vi "SimpleHEAT3.vi"() -> ()   [LabVIEW 2020]
uses:
  Control 2.ctl
  rga_lv_85/SRSRGA85.llb/SRSRGAo RefNum.ctl
  <vilib>/Utility/miscctls.llb/LVRowAndColumnTypeDef.ctl
  <vilib>/Modbus/master/Create Master Instance (TCP).vi
  <vilib>/Utility/config.llb/Read Key (String).vi
  <vilib>/Utility/config.llb/Write Key (String).vi
  <vilib>/Modbus/master/Modbus Master.lvclass
  <vilib>/Utility/config.llb/NI_LVConfig.lvlib
panel:
  in  "stop":bool
  out "Remote:":bool
  out "heat_LastData":dbl[](array[numeric])
  out "HEAT start time":timestamp=timestamp(3621395400.2120705 s since 1904-01-01)
  out "Boolean":T1=TRUE
  out "stopped_loops":bool=TRUE
  in  "Tab Control":T2(tab)
  out "Uc Act.: 2":dbl caption="Uc Act.:" format="%#_g V"
  out "Ic Act.: 2":dbl caption="Ic Act.:" format="%#_g A"
  out "Ue Act.: 2":dbl caption="Ue Act.:" format="%#_g V"
  out "Ie Act.: 2":dbl caption="Ie Act.:" format="%#_g mA"
  out "Text Ring 6":u16(ring) items=["K"=1, "C"=0]
  out "Text Ring 5":u16(ring) items=["C/s", "C/m", "C/h"]
  out "Act. Ramp:":dbl=1.0
  in  "Regulation TYpe":bool caption="Regulation Type:"
  in  "Target Ue [V]:":dbl=500.0
  in  "Target Ic [A]:":dbl=2.0
  in  "PID Output:":bool caption="PID Output Signal:"
  in  "Heating Mode:":bool
  out "Text Ring 3":u16(ring) items=["C/s", "C/m", "C/h"]
  out "Interlock:":bool
  out "Operate:":bool
  out "Text Ring":u16(ring) items=["K"=1, "C"=0]
  in  "OperateButton":bool caption="Operate:"
  out "Act. Temp:":dbl=24.100000000000023
  out "Act. P":dbl=100.0
  out "Act. I":dbl=50.0
  out "Act. D":dbl=1.0
  in  "Target Temp:":dbl=10.0
  in  "Target Ramp:":dbl=1.0
  out "Act. Setpoint:":dbl=21.55000000000001
  out "Text Ring 2":u16(ring) items=["K"=1, "C"=0]
  out "RES active:":bool
  out "EB active:":bool
  in  "Ramp unit:":u16(ring)=1 items=["/s", "/m", "/h"]
  in  "Temp. unit:":u16(ring) items=["K"=1, "C"=0]
  in  "Channel:":u16(ring)=7 items=["D1"=9, "D2"=11, "RTD"=13, "TC1"=5, "TC2"=7]
  in  "clean":bool
  out "Operate status::":bool[](array[boolean])=[FALSE, FALSE, FALSE, FALSE, FALSE, TRUE, TRUE, TRUE, FALSE, FALSE, FALSE, TRUE, FALSE, FALSE, FALSE, FALSE]
  out "Uc Act.:":dbl
  out "Ic Act.:":dbl
  out "Uc Act.:":dbl
  out "Ic Act.:":dbl
  out "Ue Act.:":dbl
  out "Ie Act.:":dbl
  in  "Ie limit [mA]:":dbl
  in  "Ue limit [V]:":dbl
  in  "Ic limit [A]:":dbl
  in  "Uc limit [V]:":dbl
  in  "Ic limit:1":dbl caption="Ic limit [A]:"
  in  "Uc limit:1":dbl caption="Uc limit [V]:"
  out "New D:":dbl=1.0
  out "New I:":dbl=50.0
  out "New P:":dbl=100.0
  in  "PID auto tab":string[][](table)
  in  "PID manual setting":string[][](table)=[["100", "50", "1"]]
  in  "Auto PID control:":bool=TRUE
  out "New PID request":bool
  out "Connected:":bool=TRUE
  in  "Reconect":bool
  out "Comunication error:":bool
  out "Loop time:":u32=499
  in  "Lock Button":bool
  in  "Address:":string="192.168.201.50"
  out "error out":T3
  # "RES:"
  # "EB:"
  # "EB:"
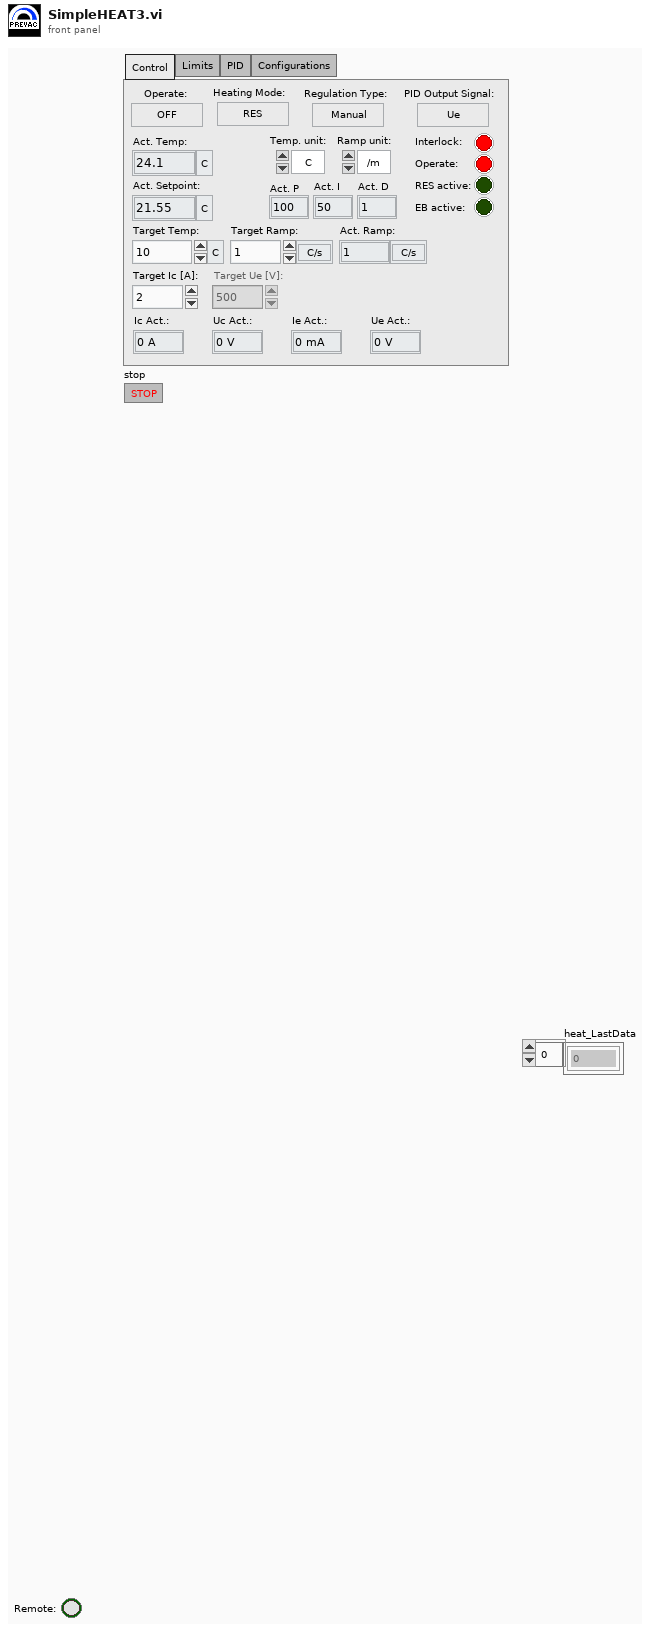
[diagram p1: front panel]
types:
  T1 = typedef "Control 2.ctl" = bool
  T2 = enum32{"Control", "Limits", "PID", "Configurations"}
  T3 = cluster{"Status:":bool, "Code:":i32, "source":string}
  T4 = typedef "SRSRGAo RefNum.ctl" = u16
  T5 = typedef "LVRowAndColumnTypeDef.ctl" = cluster{"Row":i32, "Column":i32}
  T6 = enum8{"Enabled", "Disabled", "Disabled and Grayed Out"}
  T7 = typedef "NI_LVConfig.lvlib/Config Data RefNum.ctl" = refnum<k1>
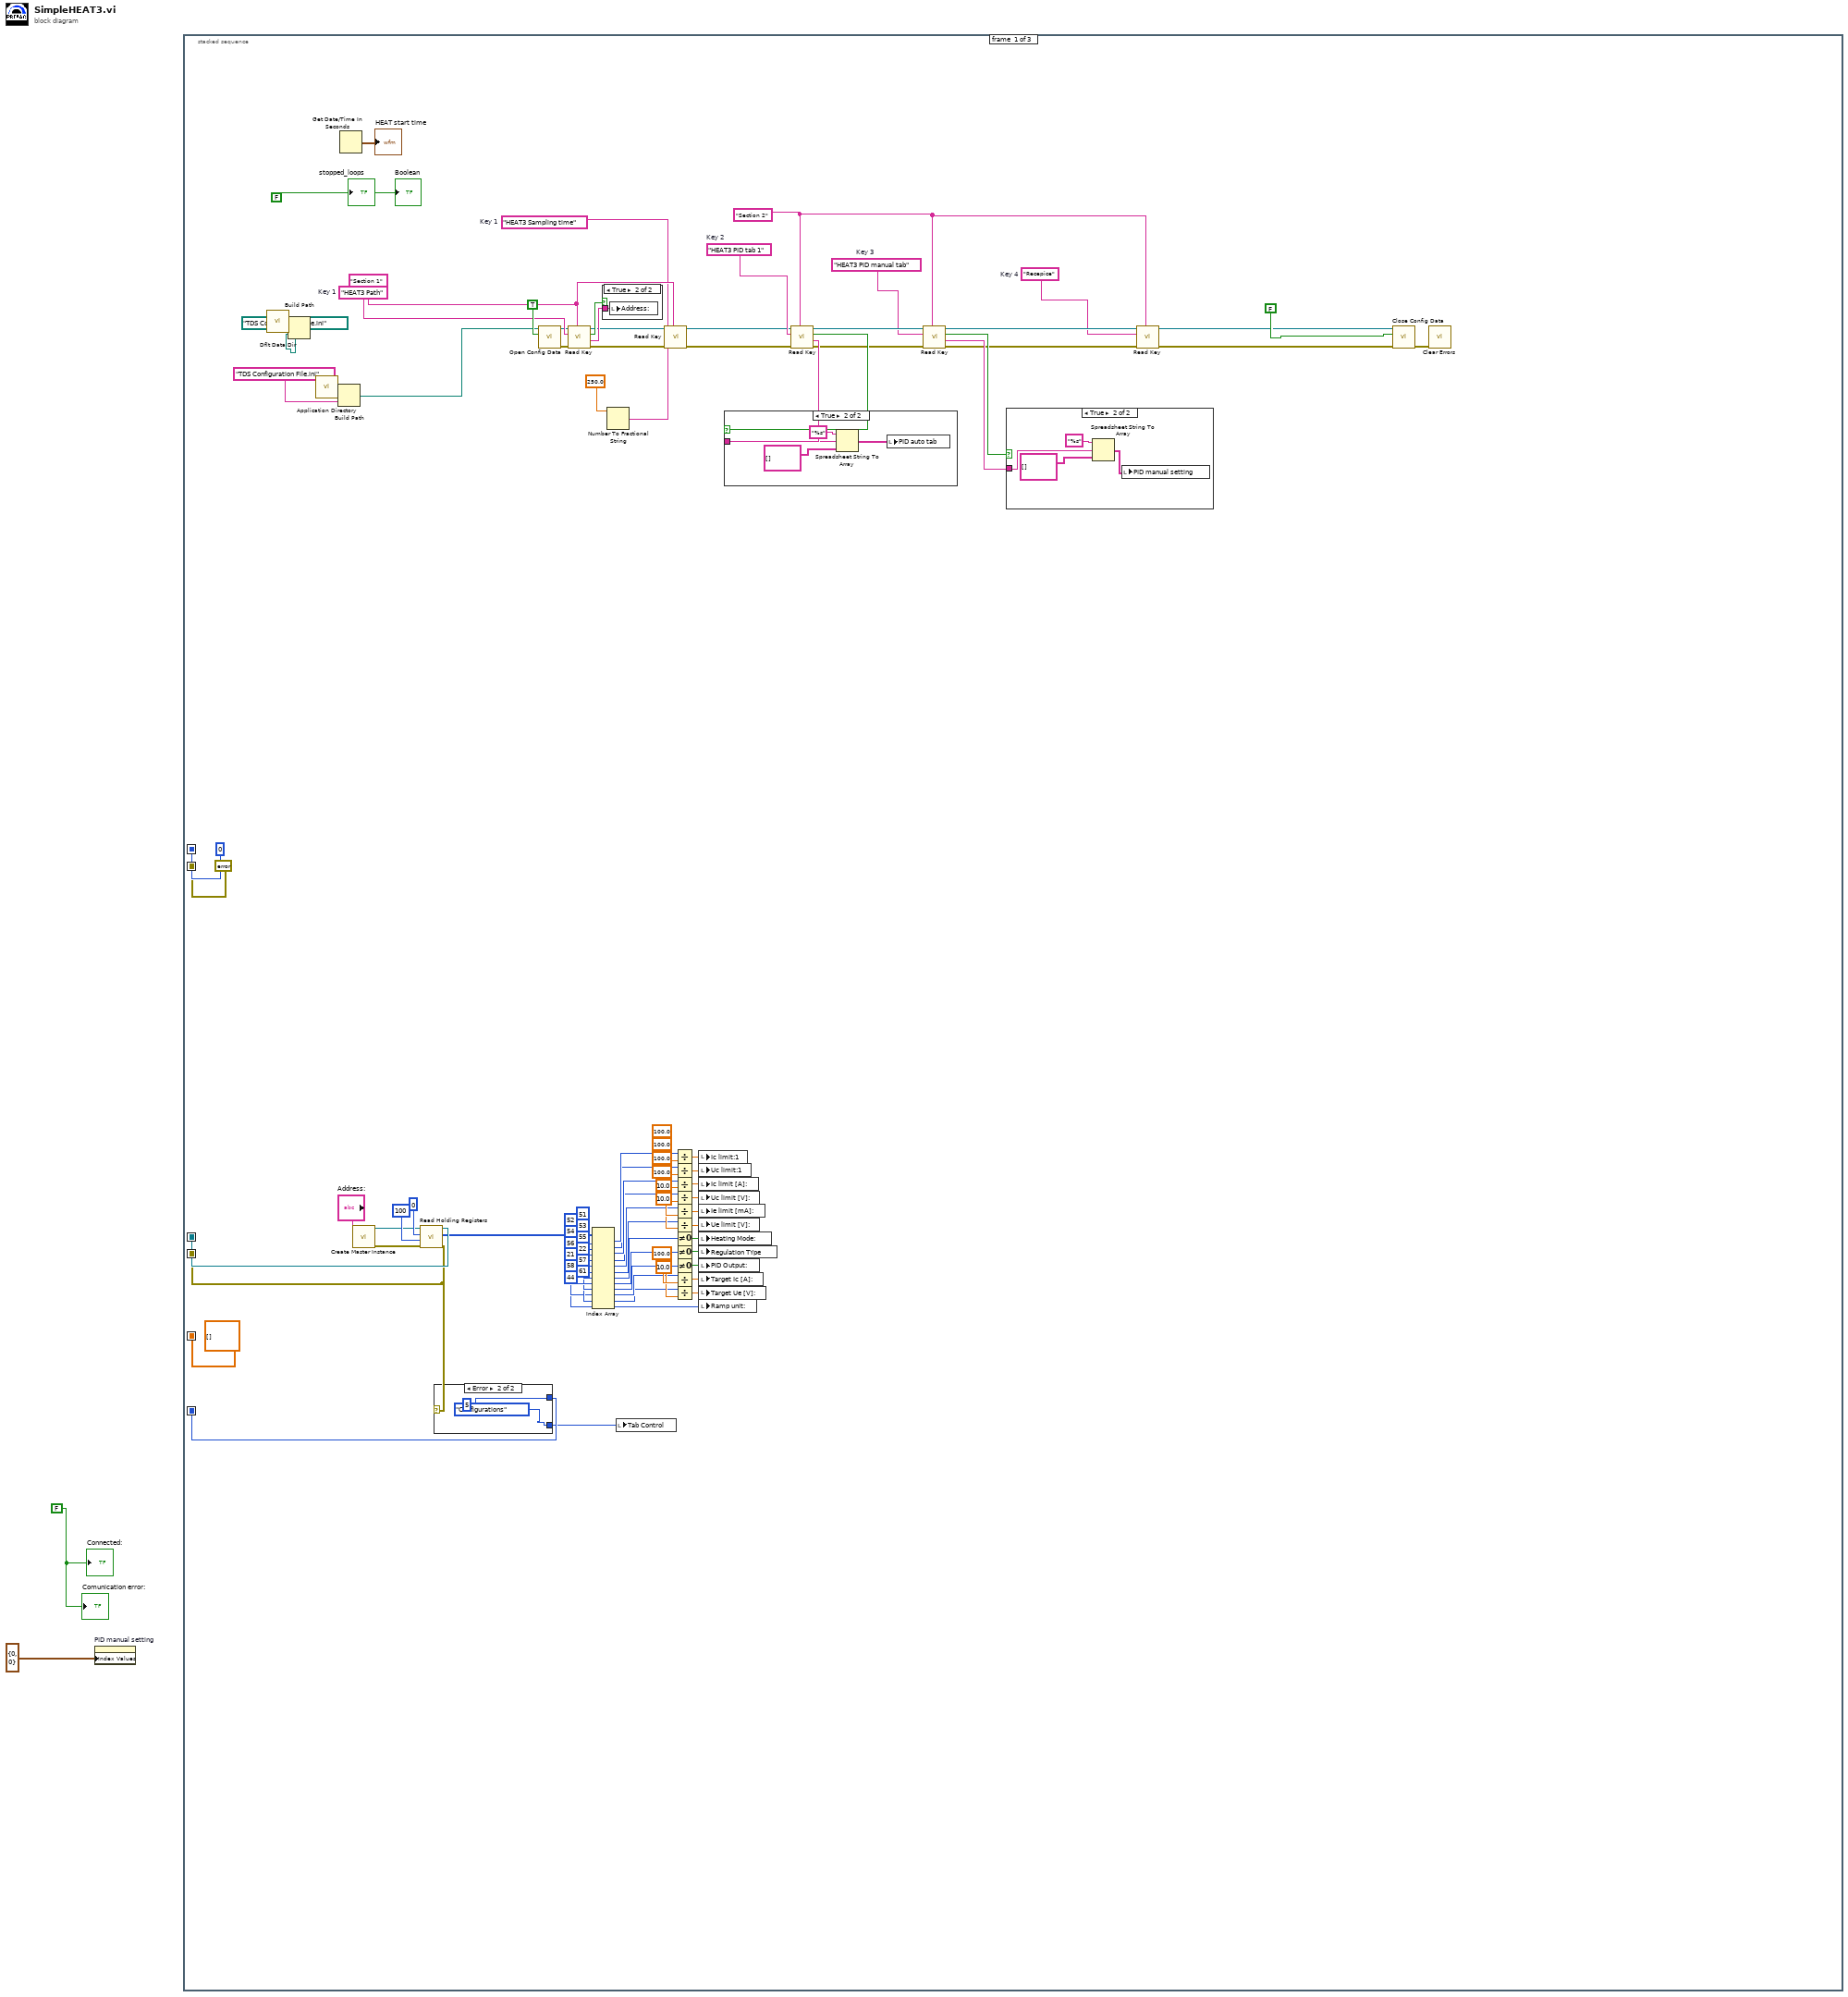
[diagram p0: block diagram]
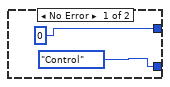
[diagram p4: hidden frame]
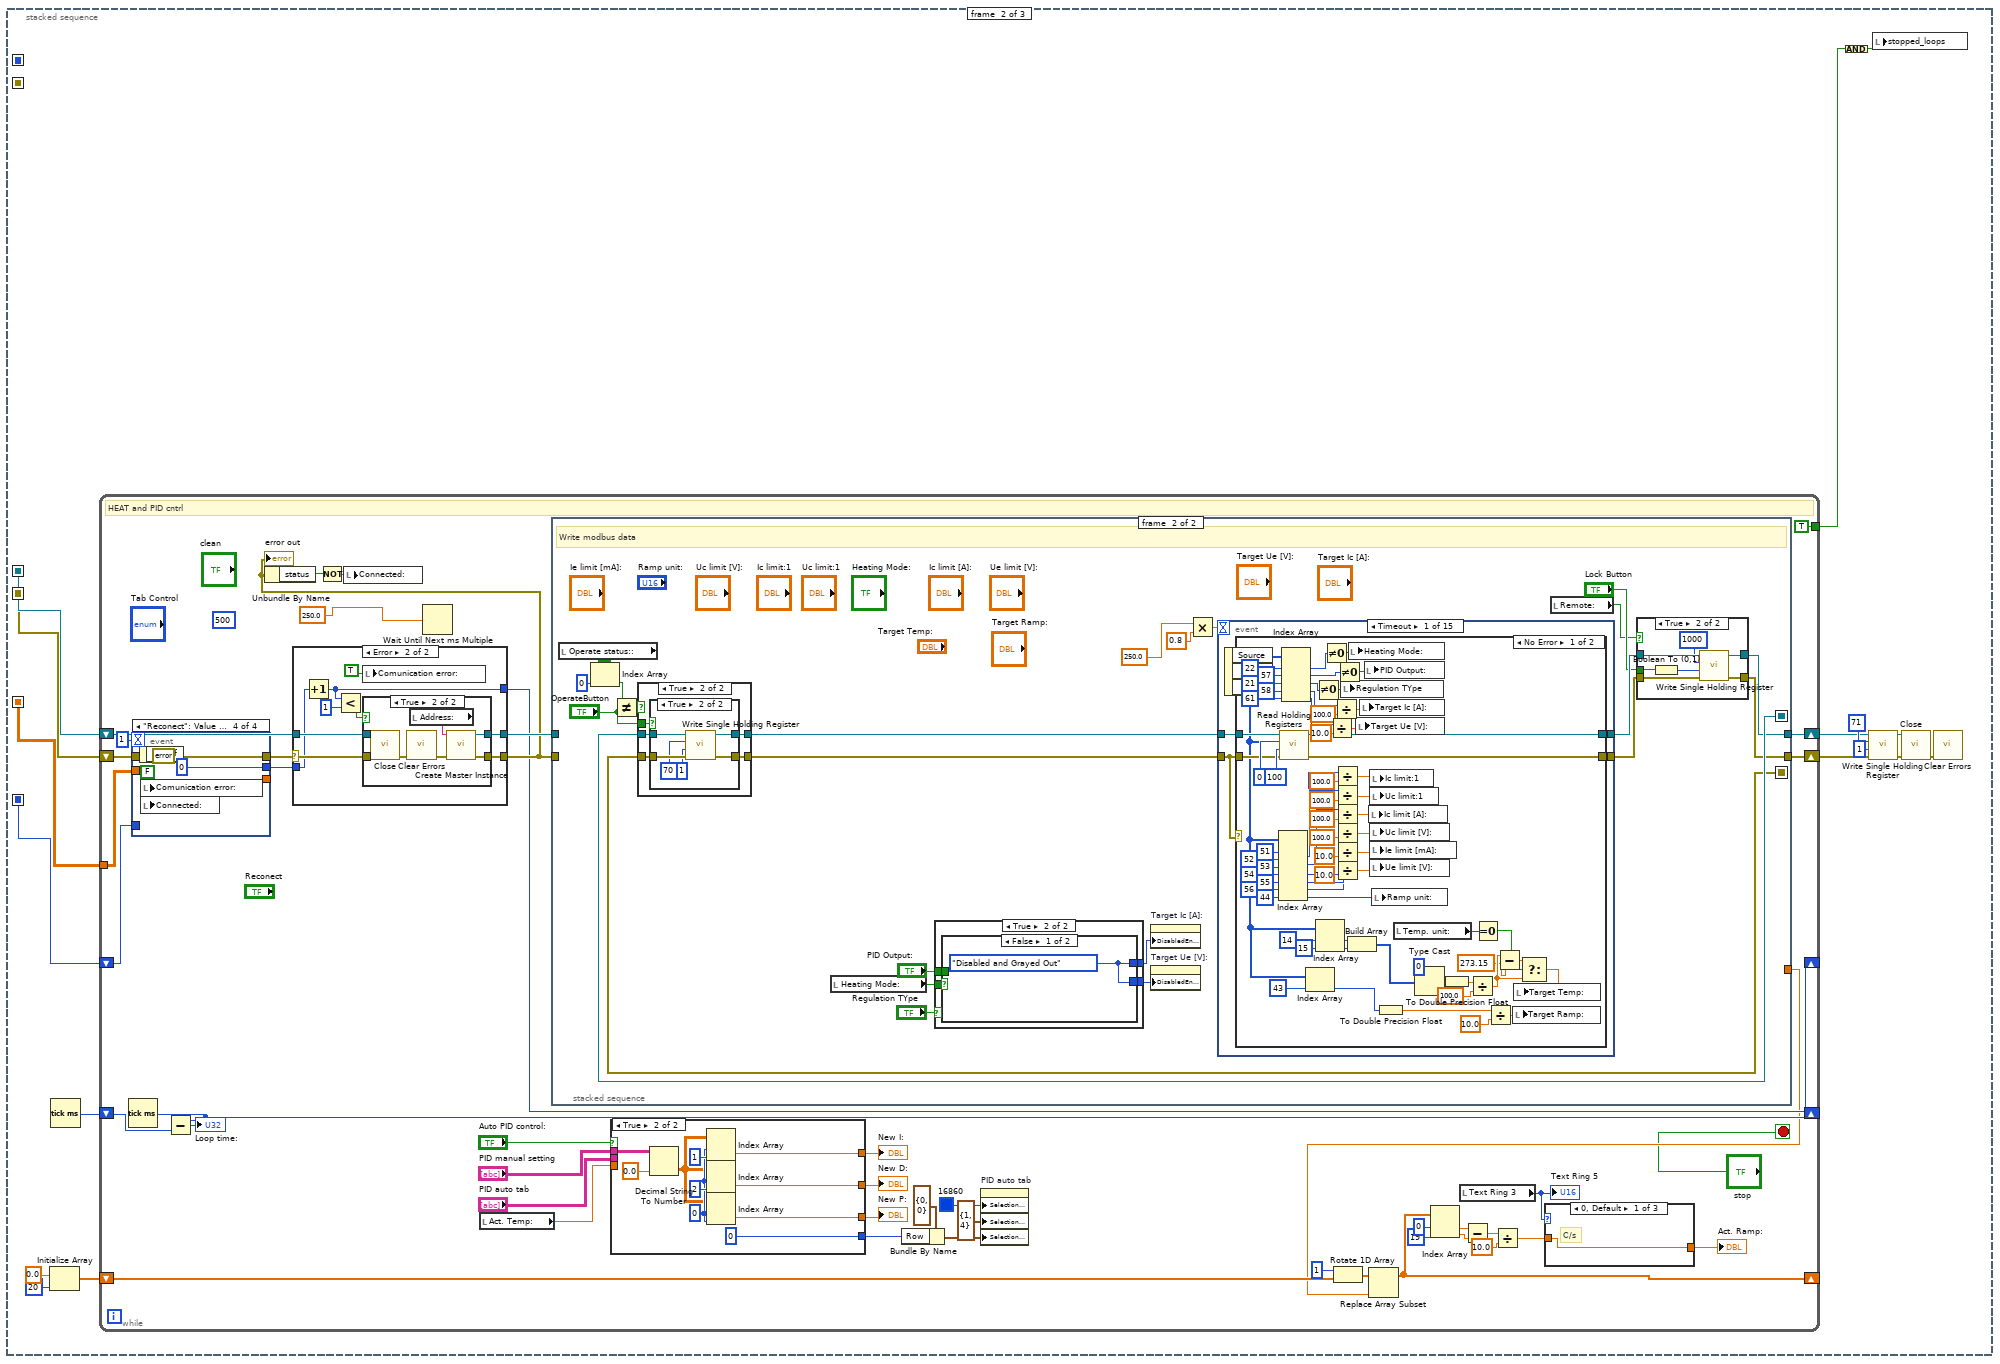
[diagram p6: hidden frame]
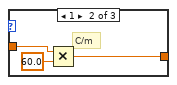
[diagram p7: hidden frame]
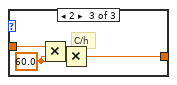
[diagram p8: hidden frame]
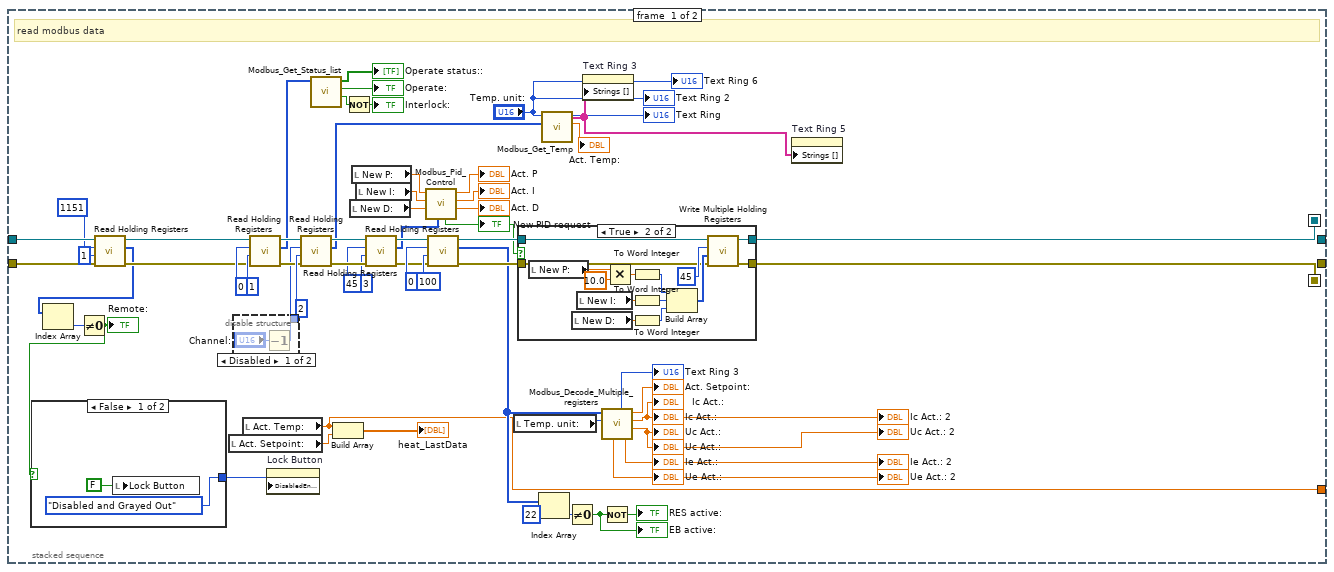
[diagram p9: hidden frame]
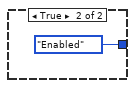
[diagram p10: hidden frame]
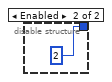
[diagram p11: hidden frame]
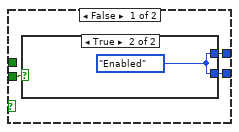
[diagram p14: hidden frame]
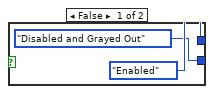
[diagram p15: hidden frame]
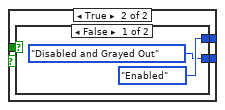
[diagram p16: hidden frame]
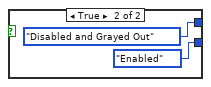
[diagram p17: hidden frame]
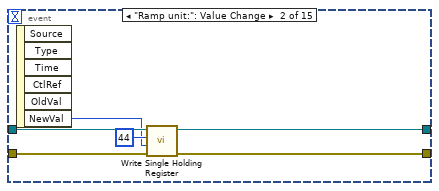
[diagram p19: hidden frame]
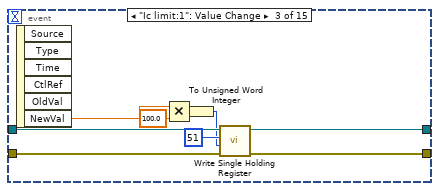
[diagram p20: hidden frame]
diagram:
  w2 = FALSE ("Connected:")
  n1 = property on="PID manual setting" class="Tbl (strict)"("Index Values"=cluster{"Row":u32, "Column":u32} {"Row"=0, "Column"=0}) -> ()  [unwired: 2 in, 2 out]
  n2 = stacked-sequence {
    seq-local: [w80 _ _] -> [_ w124 _]
    seq-local: [w33 _ _] -> [_ w123 _]
    seq-local: [dbl[][] [] _ _] -> [_ w110 _]
    seq-local: [T4 0 ("SRSRGA Refnum") _ _] -> [_ _ _]
    seq-local: [errorcluster {"status"=FALSE, "code"=0, "source"=""} ("error out") _ _] -> [_ _ _]
    seq-local: [w32 _ _] -> [_ w115 _]
    frame #0 {
      w9 = "HEAT3 Sampling time"  # Key 1
      w19 = "Recepice"  # Key 4
      w26 = "HEAT3 PID manual tab"  # Key 3
      w31 = "HEAT3 PID tab 1"  # Key 2
      w18 = "Section 2" ("section")
      w87 = "HEAT3 Path"  # Key 1
      w10 = "Section 1" ("section")
      w17 = FALSE ("Boolean")
      n3 = call <vilib>:"Dflt Data Dir.vi"() -> ("App:Default Data Directory"=w92:path)
      n4 = Build Path(base path=w92, name or relative path=path "TDS Configuration File.ini" ("default name")) -> ()  [unwired: 1 out]
      n5 = call <vilib>:"Application Directory.vi"() -> ("Application Directory"=w14:path)
      n6 = Build Path(base path=w14, name or relative path="TDS Configuration File.ini") -> (appended path=w13:path)
      n7 = Get Date/Time In Seconds() -> (seconds since 1Jan1904=→"HEAT start time":timestamp)
      n8 = call-poly <vilib>:"Create Master Instance.vi"("address"="Address:") -> ("error out"=w81:errorcluster, "TCP master instance"=w82:refnum<class "Modbus Master.lvclass">)  [unwired: 9 in]
      n9 = call-dynamic "Read Holding Registers.vi"("error in (no error)"=w81, "number of holding registers"=u16 100, "starting address"=u16 0, "Modbus master in"=w82) -> ("error out"=w33:errorcluster, "register values"=w75:u16[], "Modbus master out"=w80:refnum<class "Modbus Master.lvclass">)  [unwired: 5 in]
      n10 = case shown="Error" w33 {
        tunnel: [0 5] -> w32
        tunnel: [T2."Control" ("Tab Control") T2."Configurations" ("Tab Control")] -> w3
        frame No Error {
        }
        frame Error {
        }
      }
      n11 = call <vilib>:"Open Config Data.vi"("create file if necessary (T)"=TRUE ("create file if necessary? (T)"), "configuration file path"=w13) -> ("error out"=w85:errorcluster, "refnum"=w86:T7)  [unwired: 7 in, 1 out]
      n12 = call-poly <vilib>:"Read Key.vi"("section"=w10, "error in (no error)"=w85, "key"=w87, "refnum"=w86) -> ("error out"=w6:errorcluster, "value"=w89:string, "found?"=w88:bool, "refnum out"=w8:T7)  [unwired: 2 in, 2 out]
      n13 = Index Array(array=w75, index #1=51 ("index"), index #2=52 ("index"), index #3=53 ("index"), index #4=54 ("index"), index #5=55 ("index"), index #6=56 ("index"), index #7=22 ("index"), index #8=21 ("index"), index #9=57 ("index"), index #10=58 ("index"), index #11=61 ("index"), index #12=44 ("index")) -> (element #1=w66:u16, element #2=w65:u16, element #3=w64:u16, element #4=w52:u16, element #5=w63:u16, element #6=w51:u16, element #7=w55:u16, element #8=w4:u16, element #9=w44:u16, element #10=w37:u16, element #11=w36:u16, element #12=w34:u16)
      n14 = case shown="True" w88 {
        tunnel: w89 -> [_ w108]
        frame False {
        }
        frame True {
          n15 = local write "Address:"(w108) -> ()
        }
      }
      n16 = Number To Fractional String(number=250.0) -> (F-format string=w11:string)  [unwired: 3 in]
      n17 = local write "Tab Control"(w3) -> ()
      n18 = call-poly <vilib>:"Read Key.vi"("section"=w10, "error in (no error)"=w6, "default value"=w11, "key"=w9, "refnum"=w8) -> ("error out"=w5:errorcluster, "refnum out"=w7:T7)  [unwired: 1 in, 4 out]
      n19 = Divide(x=w66, y=100.0) -> (x/y=w62:dbl)
      n20 = Divide(x=w65, y=100.0) -> (x/y=w61:dbl)
      n21 = Divide(x=w64, y=100.0) -> (x/y=w60:dbl)
      n22 = Divide(x=w52, y=100.0) -> (x/y=w59:dbl)
      n23 = Divide(x=w63, y=10.0) -> (x/y=w58:dbl)
      n24 = Divide(x=w51, y=10.0) -> (x/y=w57:dbl)
      n25 = Not Equal To 0?(x=w55) -> (x != 0?=w54:bool)
      n26 = Not Equal To 0?(x=w4) -> (x != 0?=w48:bool)
      n27 = Not Equal To 0?(x=w44) -> (x != 0?=w47:bool)
      n28 = Divide(x=w37, y=100.0) -> (x/y=w41:dbl)
      n29 = Divide(x=w36, y=10.0) -> (x/y=w40:dbl)
      n30 = local write "Ic limit:1"(w62) -> ()
      n31 = local write "Uc limit:1"(w61) -> ()
      n32 = local write "Ic limit [A]:"(w60) -> ()
      n33 = local write "Uc limit [V]:"(w59) -> ()
      n34 = local write "Ie limit [mA]:"(w58) -> ()
      n35 = local write "Ue limit [V]:"(w57) -> ()
      n36 = local write "Heating Mode:"(w54) -> ()
      n37 = local write "Regulation TYpe"(w48) -> ()
      n38 = local write "PID Output:"(w47) -> ()
      n39 = local write "Target Ic [A]:"(w41) -> ()
      n40 = local write "Target Ue [V]:"(w40) -> ()
      n41 = local write "Ramp unit:"(w34) -> ()
      n42 = call-poly <vilib>:"Read Key.vi"("section"=w18, "error in (no error)"=w5, "key"=w31, "refnum"=w7) -> ("error out"=w27:errorcluster, "value"=w29:string, "found?"=w30:bool, "refnum out"=w28:T7)  [unwired: 2 in, 2 out]
      n43 = case shown="True" w30 {
        tunnel: w29 -> [_ w103]
        frame False {
        }
        frame True {
          n44 = Spreadsheet String To Array(format string="%s", spreadsheet string=w103, array type (2D Dbl)=string[][] [] ("PID auto tab")) -> (array=w100:string[][])  [unwired: 1 in]
          n45 = local write "PID auto tab"(w100) -> ()
        }
      }
      n46 = call-poly <vilib>:"Read Key.vi"("section"=w18, "error in (no error)"=w27, "key"=w26, "refnum"=w28) -> ("error out"=w23:errorcluster, "value"=w24:string, "found?"=w25:bool, "refnum out"=w21:T7)  [unwired: 2 in, 2 out]
      n47 = case shown="True" w25 {
        tunnel: w24 -> [_ w97]
        frame False {
        }
        frame True {
          n48 = Spreadsheet String To Array(format string="%s", spreadsheet string=w97, array type (2D Dbl)=string[][] [] ("PID auto tab")) -> (array=w96:string[][])  [unwired: 1 in]
          n49 = local write "PID manual setting"(w96) -> ()
        }
      }
      n50 = call-poly <vilib>:"Read Key.vi"("section"=w18, "error in (no error)"=w23, "key"=w19, "refnum"=w21) -> ("error out"=w22:errorcluster, "refnum out"=w20:T7)  [unwired: 2 in, 4 out]
      n51 = call <vilib>:"Close Config Data.vi"("error in (no error)"=w22, "write file if changed (T)"=FALSE ("write configuration file? (T)"), "refnum"=w20) -> ("error out"=w16:errorcluster)  [unwired: 8 out]
      n52 = call <vilib>:"Clear Errors.vi"("error in (no error)"=w16) -> ()  [unwired: 5 in, 2 out]
      "stopped_loops" <- w17
      "Boolean" <- w17
    }
    frame #1 {
      n53 = Initialize Array(0.0 ("element"), 20 ("dimension size")) -> (w112:dbl[])
      n54 = Tick Count (ms)() -> (millisecond timer value=w111:u32)
      n55 = while {
        tunnel: [TRUE] -> w116
        shift-right: [w156] -> w119
        shift-left: w123 -> [w149]
        shift-right: [w159] -> w120
        shift-left: w124 -> [w158]
        shift-right: [w153] -> _
        shift-left: w111 -> [w152]
        shift-right: [w142] -> _
        shift-left: w115 -> [w147]
        tunnel: w110 -> [w154]
        shift-right: [w138] -> _
        shift-left: w112 -> [w141]
        stop <- "stop" stop-if-true
        (unwired) u32 500 ("millisecond multiple")
        # "HEAT and PID cntrl"
        n56 = Tick Count (ms)() -> (millisecond timer value=w153:u32)
        n57 = event shown="[3] \"Reconect\": Value Change" {
          selector: _ -> [_ _ _ _]
          dyn-events: _ -> [_ _ _ _]
          timeout: 1 -> [_ _ _ _]
          tunnel: w154 -> [w540 _ _ _]
          tunnel: [w538 dbl[][] [] _ _] -> _
          tunnel: [w537 w543 errorcluster {"status"=TRUE, "code"=0, "source"="Connect to\nnew IP addres"} ("error constant") errorcluster {"status"=TRUE, "code"=0, "source"="Rconnecting"} ("error constant")] -> w148
          tunnel: w149 -> [w537 w543 _ _]
          tunnel: [w536 w542 0 0] -> w146
          tunnel: w147 -> [w536 w542 _ _]
          event Timeout {
            n58 = event-data() -> ()  [unwired: 1 in, 1 out]
            n59 = Select(t=w540, s=FALSE ("build array of data?"), f=dbl[][] []) -> (s? t:f=w538:dbl[][])
          }
          event "clean": Value Change {
            n60 = event-data() -> ()  [unwired: 1 in, 1 out]
            n61 = Get Date/Time In Seconds() -> (seconds since 1Jan1904=w544:timestamp)
            n62 = local write "HEAT start time"(w544) -> ()
            n63 = local write "clean"(FALSE ("clc graph")) -> ()
          }
          event "Address:": Value Change {
            n64 = event-data() -> ()  [unwired: 1 in, 1 out]
          }
          event "Reconect": Value Change {
            w549 = FALSE ("Connected:")
            n65 = event-data() -> ()  [unwired: 1 in, 1 out]
            n66 = local write "Comunication error:"(w549) -> ()
            n67 = local write "Connected:"(w549) -> ()
          }
        }
        n68 = Subtract(x=w153, y=w152) -> (x-y=→"Loop time:":u32)
        n69 = case shown="Error" w148 {
          selector: w148 -> [w556 w565]
          tunnel: [w556 w562] -> w144
          tunnel: w158 -> [w555 w564]
          tunnel: [w555 w563] -> w157
          tunnel: w146 -> [_ w560]
          tunnel: [0 w559] -> w142
          frame No Error {
            w552 = FALSE
            n70 = Not(x=w552) -> (.not. x?=w553:bool)
            n71 = local write "Comunication error:"(w552) -> ()
            n72 = local write "Connected:"(w553) -> ()
          }
          frame Error {
            n73 = Increment(x=w560) -> (x+1=w559:i32)
            n74 = Less?(x=w559, y=1) -> (x < y?=w558:bool)
            n75 = local write "Comunication error:"(TRUE) -> ()
            n76 = case shown="True" w558 {
              tunnel: w565 -> [w566 w574]
              tunnel: w564 -> [w567 w573]
              tunnel: [w567 w571] -> w563
              tunnel: [w566 w570] -> w562
              frame False {
              }
              frame True {
                n77 = call-dynamic "Close.vi"("error in (no error)"=w574, "Modbus master in"=w573) -> ("error out"=w569:errorcluster)  [unwired: 9 in]
                n78 = call <vilib>:"Clear Errors.vi"("error in (no error)"=w569) -> ("error out"=w568:errorcluster)  [unwired: 5 in, 1 out]
                n79 = local read "Address:"() -> (w572:string)
                n80 = call-poly <vilib>:"Create Master Instance.vi"("error in (no error)"=w568, "address"=w572) -> ("error out"=w570:errorcluster, "TCP master instance"=w571:refnum<class "Modbus Master.lvclass">)  [unwired: 8 in]
              }
            }
          }
        }
        "error out" <- w144
        n81 = Unbundle By Name(w144) -> ("status"=w145:bool)
        n82 = Not(x=w145) -> (.not. x?=w143:bool)
        n83 = local write "Connected:"(w143) -> ()
        n84 = Wait Until Next ms Multiple(millisecond multiple=250.0 ("y")) -> ()  [unwired: 1 out]
        n85 = local read "Act. Temp:"() -> (w160:dbl)
        n86 = stacked-sequence {
          seq-local: [w200 _] -> [_ w279]
          seq-local: [w199 _] -> [_ w278]
          tunnel: w157 -> [w198 _]
          tunnel: w144 -> [w197 _]
          tunnel: [_ w271] -> w159
          tunnel: [_ w269] -> w156
          tunnel: [w188 _] -> w128
          frame #0 {
            # "read modbus data"
            n87 = call-dynamic "Read Holding Registers.vi"("error in (no error)"=w197, "number of holding registers"=u16 1, "starting address"=u16 1151, "Modbus master in"=w198) -> ("error out"=w195:errorcluster, "register values"=w189:u16[], "Modbus master out"=w196:refnum<class "Modbus Master.lvclass">)  [unwired: 5 in]
            n88 = Index Array(array=w189) -> (element=w190:u16)  [unwired: 1 in]
            n89 = Not Equal To 0?(x=w190) -> (x != 0?=w191:bool)
            "Remote:" <- w191
            n90 = case shown="False" w191 {
              tunnel: [T6."Disabled and Grayed Out" ("Disabled") T6."Enabled" ("Disabled")] -> w192
              frame False {
                n91 = local write "Lock Button"(FALSE ("Lock Button")) -> ()
              }
              frame True {
              }
            }
            n92 = local read "Act. Setpoint:"() -> (w213:dbl)
            n93 = disable-structure shown="Disabled" {
              disable-tunnel: [w243 u16 2] -> w218
              frame Disabled {
                n94 = Decrement(x="Channel:") -> (x-1=w243:u16)
              }
              frame Enabled {
              }
            }
            n95 = local read "Act. Temp:"() -> (w188:dbl)
            n96 = call-dynamic "Read Holding Registers.vi"("error in (no error)"=w195, "number of holding registers"=u16 1, "starting address"=u16 0, "Modbus master in"=w196) -> ("error out"=w231:errorcluster, "register values"=w206:u16[], "Modbus master out"=w232:refnum<class "Modbus Master.lvclass">)  [unwired: 5 in]
            n97 = property on="Lock Button" class="Bool (strict)"("DisabledEnum"=w192) -> ()  [unwired: 2 in, 2 out]
            n98 = call-dynamic "Read Holding Registers.vi"("error in (no error)"=w231, "number of holding registers"=u16 2, "starting address"=w218, "Modbus master in"=w232) -> ("error out"=w237:errorcluster, "register values"=w216:u16[], "Modbus master out"=w238:refnum<class "Modbus Master.lvclass">)  [unwired: 5 in]
            n99 = call "Modbus_Get_Status_list.vi"("register values"=w206) -> ("Boolean"=w210:bool, "Boolean 2"=→"Operate:":bool, "Boolean array"=→"Operate status::":bool[])  [unwired: 8 in]
            n100 = Build Array(w188, w213) -> (→"heat_LastData":dbl[])
            n101 = Not(x=w210) -> (.not. x?=→"Interlock:":bool)
            n102 = local read "New D:"() -> (w227:dbl)
            n103 = local read "New P:"() -> (w225:dbl)
            n104 = local read "New I:"() -> (w229:dbl)
            n105 = call-dynamic "Read Holding Registers.vi"("error in (no error)"=w237, "number of holding registers"=u16 3, "starting address"=u16 45, "Modbus master in"=w238) -> ("error out"=w220:errorcluster, "register values"=w208:u16[], "Modbus master out"=w222:refnum<class "Modbus Master.lvclass">)  [unwired: 5 in]
            n106 = call "Modbus_Pid_Control.vi"("register values"=w208, "new D"=w227, "new I"=w229, "new P"=w225) -> ("Numeric"=→"Act. D":dbl, "Numeric 2"=→"Act. I":dbl, "Numeric 3"=→"Act. P":dbl, "Boolean"=w207:bool)  [unwired: 4 in]
            "New PID request" <- w207
            n107 = call-dynamic "Read Holding Registers.vi"("error in (no error)"=w220, "number of holding registers"=u16 100, "starting address"=u16 0, "Modbus master in"=w222) -> ("error out"=w219:errorcluster, "register values"=w201:u16[], "Modbus master out"=w221:refnum<class "Modbus Master.lvclass">)  [unwired: 5 in]
            n108 = local read "Temp. unit:"() -> (w215:u16)
            n109 = case shown="True" w207 {
              tunnel: w221 -> [w246 w251]
              tunnel: w219 -> [w247 w250]
              tunnel: [w246 w249] -> w200
              tunnel: [w247 w248] -> w199
              frame False {
              }
              frame True {
                n110 = local read "New P:"() -> (w259:dbl)
                n111 = local read "New D:"() -> (w261:dbl)
                n112 = local read "New I:"() -> (w260:dbl)
                n113 = Multiply(x=w259, y=10.0) -> (x*y=w255:dbl)
                n114 = To Word Integer(number=w255) -> (16bit integer=w256:i16)
                n115 = To Word Integer(number=w260) -> (16bit integer=w257:i16)
                n116 = To Word Integer(number=w261) -> (16bit integer=w258:i16)
                n117 = Build Array(w256, w257, w258) -> (w252:i16[])
                n118 = call-dynamic "Write Multiple Holding Registers.vi"("error in (no error)"=w250, "holding register values"=w252, "starting address"=u16 45, "Modbus master in"=w251) -> ("error out"=w248:errorcluster, "Modbus master out"=w249:refnum<class "Modbus Master.lvclass">)  [unwired: 6 in]
              }
            }
            n119 = Index Array(array=w201, index=22) -> (element=w204:u16)
            n120 = call "Modbus_Get_Temp.vi"("register values"=w216, "Temp. unit:"="Temp. unit:") -> ("Numeric"=→"Act. Temp:":dbl, "Strings []"=w185:string[])  [unwired: 8 in]
            n121 = Not Equal To 0?(x=w204) -> (x != 0?=w203:bool)
            "EB active:" <- w203
            n122 = property on="Text Ring 3" class="Ring (strict)"("Strings []"=w185) -> ()  [unwired: 2 in, 2 out]
            n123 = call "Modbus_Decode_Multiple_registers.vi"("Temp. unit:"=w215, "register values"=w201) -> ("Numeric 3"=→"Uc Act.:" →"Uc Act.:" →"Uc Act.: 2":dbl, "Numeric 4"=→"Ic Act.:" →"Ic Act.:" →"Ic Act.: 2":dbl, "Numeric 5"=→"Act. Setpoint:":dbl, "Numeric 2"=→"Ie Act.:" →"Ie Act.: 2":dbl, "register"=→"Text Ring 3":u16, "Numeric"=→"Ue Act.:" →"Ue Act.: 2":dbl)  [unwired: 4 in]
            n124 = Not(x=w203) -> (.not. x?=→"RES active:":bool)
            n125 = property on="Text Ring 5" class="Ring (strict)"("Strings []"=w185) -> ()  [unwired: 2 in, 2 out]
            "Text Ring" <- "Temp. unit:"
            "Text Ring 2" <- "Temp. unit:"
            "Text Ring 6" <- "Temp. unit:"
          }
          frame #1 {
            # "Write modbus data"
            n126 = local read "Operate status::"() -> (w284:bool[])
            n127 = Index Array(array=w284, index=0) -> (element=w282:bool)
            n128 = Not Equal?(x=w282, y="OperateButton") -> (x != y?=w281:bool)
            n129 = case shown="True" w281 {
              tunnel: w279 -> [w518 w523]
              tunnel: w278 -> [w517 w522]
              tunnel: [w518 w521] -> w264
              tunnel: [w517 w520] -> w263
              tunnel: "OperateButton" -> [_ w519]
              frame False {
              }
              frame True {
                n130 = case shown="True" w519 {
                  tunnel: w523 -> [w527 w535]
                  tunnel: w522 -> [w526 w534]
                  tunnel: [w525 w533] -> w521
                  tunnel: [w524 w532] -> w520
                  frame False {
                    n131 = call-dynamic "Write Single Holding Register.vi"("error in (no error)"=w526, "holding register value"=u16 1, "address"=u16 71, "Modbus master in"=w527) -> ("error out"=w524:errorcluster, "Modbus master out"=w525:refnum<class "Modbus Master.lvclass">)  [unwired: 6 in]
                  }
                  frame True {
                    n132 = call-dynamic "Write Single Holding Register.vi"("error in (no error)"=w534, "holding register value"=u16 1, "address"=u16 70, "Modbus master in"=w535) -> ("error out"=w532:errorcluster, "Modbus master out"=w533:refnum<class "Modbus Master.lvclass">)  [unwired: 6 in]
                  }
                }
              }
            }
            n133 = local read "Heating Mode:"() -> (w274:bool)
            n134 = case shown="True" "Regulation TYpe" {
              tunnel: [w295 w303] -> w276
              tunnel: [w294 w302] -> w275
              tunnel: w274 -> [w296 w301]
              tunnel: "PID Output:" -> [_ w300]
              frame False {
                n135 = case shown="True" w296 {
                  tunnel: [T6."Enabled" ("Disabled") w299] -> w295
                  tunnel: [T6."Disabled and Grayed Out" ("Disabled") w299] -> w294
                  frame False {
                  }
                  frame True {
                    w299 = T6."Enabled" ("Disabled")
                  }
                }
              }
              frame True {
                n136 = case shown="False" w301 {
                  tunnel: [w304 w306] -> w303
                  tunnel: [w304 w305] -> w302
                  tunnel: w300 -> [_ w307]
                  frame False {
                    w304 = T6."Disabled and Grayed Out" ("Disabled")
                  }
                  frame True {
                    n137 = case shown="False" w307 {
                      tunnel: [T6."Enabled" ("Disabled") T6."Disabled and Grayed Out" ("Disabled")] -> w306
                      tunnel: [T6."Disabled and Grayed Out" ("Disabled") T6."Enabled" ("Disabled")] -> w305
                      frame False {
                      }
                      frame True {
                      }
                    }
                  }
                }
              }
            }
            n138 = property on="Target Ic [A]:" class="DigNum (strict)"("DisabledEnum"=w276) -> ()  [unwired: 2 in, 2 out]
            n139 = property on="Target Ue [V]:" class="DigNum (strict)"("DisabledEnum"=w275) -> ()  [unwired: 2 in, 2 out]
            n140 = Multiply(x=250.0 ("y"), y=0.8) -> (x*y=w265:dbl)
            n141 = event shown="[0] Timeout" {
              selector: _ -> [_ _ _ _ _ _ _ _ _ _ _ _ _ _ _]
              dyn-events: _ -> [_ _ _ _ _ _ _ _ _ _ _ _ _ _ _]
              timeout: w265 -> [_ _ _ _ _ _ _ _ _ _ _ _ _ _ _]
              tunnel: w264 -> [w315 w390 w399 w408 w417 w426 w435 w444 w453 w462 w470 w478 w486 w505 w513]
              tunnel: [w313 w391 w400 w409 w418 w427 w436 w445 w454 w463 w471 w479 w487 w502 w514] -> w270
              tunnel: w263 -> [w312 w389 w398 w407 w416 w425 w434 w443 w452 w461 w469 w477 w485 w504 w512]
              tunnel: [w314 w392 w401 w410 w419 w428 w437 w446 w455 w464 w472 w480 w488 w503 w515] -> w272
              event Timeout {
                n142 = event-data() -> ()  [unwired: 1 in, 3 out]
                n143 = case shown="No Error" w312 {
                  tunnel: w315 -> [w366 w387]
                  tunnel: w312 -> [w365 w386]
                  tunnel: [w364 w387] -> w314
                  tunnel: [w363 w386] -> w313
                  frame No Error {
                    n144 = call-dynamic "Read Holding Registers.vi"("error in (no error)"=w365, "number of holding registers"=u16 100, "starting address"=u16 0, "Modbus master in"=w366) -> ("error out"=w363:errorcluster, "register values"=w320:u16[], "Modbus master out"=w364:refnum<class "Modbus Master.lvclass">)  [unwired: 5 in]
                    n145 = Index Array(array=w320, index #1=51 ("index"), index #2=52 ("index"), index #3=53 ("index"), index #4=54 ("index"), index #5=55 ("index"), index #6=56 ("index"), index #7=u16 44 ("address")) -> (element #1=w358:u16, element #2=w359:u16, element #3=w360:u16, element #4=w362:u16, element #5=w361:u16, element #6=w338:u16, element #7=w337:u16)
                    n146 = Index Array(array=w320, index #1=u16 22 ("address"), index #2=u16 57 ("address"), index #3=u16 21 ("address"), index #4=u16 58 ("address"), index #5=61 ("index")) -> (element #1=w384:u16, element #2=w381:u16, element #3=w378:u16, element #4=w375:u16, element #5=w371:u16)
                    n147 = Index Array(array=w320, index=u16 43 ("address")) -> (element=w318:u16)
                    n148 = Not Equal To 0?(x=w378) -> (x != 0?=w379:bool)
                    n149 = Index Array(array=w320, index #1=u16 14 ("address"), index #2=u16 15 ("address")) -> (element #1=w334:u16, element #2=w333:u16)
                    n150 = Not Equal To 0?(x=w384) -> (x != 0?=w385:bool)
                    n151 = Divide(x=w371, y=10.0) -> (x/y=w373:dbl)
                    n152 = Divide(x=w375, y=100.0) -> (x/y=w376:dbl)
                    n153 = Divide(x=w358, y=100.0) -> (x/y=w340:dbl)
                    n154 = Divide(x=w359, y=100.0) -> (x/y=w341:dbl)
                    n155 = Divide(x=w360, y=100.0) -> (x/y=w342:dbl)
                    n156 = Divide(x=w362, y=100.0) -> (x/y=w343:dbl)
                    n157 = Divide(x=w361, y=10.0) -> (x/y=w344:dbl)
                    n158 = Divide(x=w338, y=10.0) -> (x/y=w345:dbl)
                    n159 = Not Equal To 0?(x=w381) -> (x != 0?=w382:bool)
                    n160 = local write "Regulation TYpe"(w379) -> ()
                    n161 = Build Array(w334, w333) -> (w322:u16[])
                    n162 = local write "Heating Mode:"(w385) -> ()
                    n163 = local write "Target Ue [V]:"(w373) -> ()
                    n164 = local write "Target Ic [A]:"(w376) -> ()
                    n165 = local write "PID Output:"(w382) -> ()
                    n166 = local write "Ic limit [A]:"(w342) -> ()
                    n167 = local write "Ic limit:1"(w340) -> ()
                    n168 = local write "Uc limit:1"(w341) -> ()
                    n169 = local write "Uc limit [V]:"(w343) -> ()
                    n170 = local write "Ie limit [mA]:"(w344) -> ()
                    n171 = local write "Ue limit [V]:"(w345) -> ()
                    n172 = local write "Ramp unit:"(w337) -> ()
                    n173 = To Double Precision Float(number=w318) -> (double precision float=w317:dbl)
                    n174 = local read "Temp. unit:"() -> (w331:u16)
                    n175 = Type Cast(type=0, x=w322) -> (*(type *) &x=w330:i32)
                    n176 = To Double Precision Float(number=w330) -> (double precision float=w329:dbl)
                    n177 = Divide(x=w329, y=100.0) -> (x/y=w328:dbl)
                    n178 = Equal To 0?(x=w331) -> (x = 0?=w326:bool)
                    n179 = Divide(x=w317, y=10.0) -> (x/y=w316:dbl)
                    n180 = Subtract(x=w328, y=273.15) -> (x-y=w327:dbl)
                    n181 = local write "Target Ramp:"(w316) -> ()
                    n182 = Select(t=w327, s=w326, f=w328) -> (s? t:f=w332:dbl)
                    n183 = local write "Target Temp:"(w332) -> ()
                  }
                  frame Error {
                  }
                }
              }
              event "Ramp unit:": Value Change {
                n184 = event-data() -> ("NewVal"=w388:u16)  [unwired: 1 in, 5 out]
                n185 = call-dynamic "Write Single Holding Register.vi"("error in (no error)"=w389, "holding register value"=w388, "address"=u16 44, "Modbus master in"=w390) -> ("error out"=w391:errorcluster, "Modbus master out"=w392:refnum<class "Modbus Master.lvclass">)  [unwired: 6 in]
              }
              event "Ic limit:1": Value Change {
                n186 = event-data() -> ("NewVal"=w395:dbl)  [unwired: 1 in, 5 out]
                n187 = Multiply(x=w395, y=100.0) -> (x*y=w397:dbl)
                n188 = To Unsigned Word Integer(number=w397) -> (unsigned 16bit integer=w394:u16)
                n189 = call-dynamic "Write Single Holding Register.vi"("error in (no error)"=w398, "holding register value"=w394, "address"=u16 51, "Modbus master in"=w399) -> ("error out"=w400:errorcluster, "Modbus master out"=w401:refnum<class "Modbus Master.lvclass">)  [unwired: 6 in]
              }
              event "Uc limit:1": Value Change {
                n190 = event-data() -> ("NewVal"=w404:dbl)  [unwired: 1 in, 5 out]
                n191 = Multiply(x=w404, y=100.0) -> (x*y=w406:dbl)
                n192 = To Unsigned Word Integer(number=w406) -> (unsigned 16bit integer=w403:u16)
                n193 = call-dynamic "Write Single Holding Register.vi"("error in (no error)"=w407, "holding register value"=w403, "address"=u16 52, "Modbus master in"=w408) -> ("error out"=w409:errorcluster, "Modbus master out"=w410:refnum<class "Modbus Master.lvclass">)  [unwired: 6 in]
              }
              event "Ic limit [A]:": Value Change {
                n194 = event-data() -> ("NewVal"=w413:dbl)  [unwired: 1 in, 5 out]
                n195 = Multiply(x=w413, y=100.0) -> (x*y=w415:dbl)
                n196 = To Unsigned Word Integer(number=w415) -> (unsigned 16bit integer=w412:u16)
                n197 = call-dynamic "Write Single Holding Register.vi"("error in (no error)"=w416, "holding register value"=w412, "address"=u16 53, "Modbus master in"=w417) -> ("error out"=w418:errorcluster, "Modbus master out"=w419:refnum<class "Modbus Master.lvclass">)  [unwired: 6 in]
              }
              event "Uc limit [V]:": Value Change {
                n198 = event-data() -> ("NewVal"=w422:dbl)  [unwired: 1 in, 5 out]
                n199 = Multiply(x=w422, y=100.0) -> (x*y=w424:dbl)
                n200 = To Unsigned Word Integer(number=w424) -> (unsigned 16bit integer=w421:u16)
                n201 = call-dynamic "Write Single Holding Register.vi"("error in (no error)"=w425, "holding register value"=w421, "address"=u16 54, "Modbus master in"=w426) -> ("error out"=w427:errorcluster, "Modbus master out"=w428:refnum<class "Modbus Master.lvclass">)  [unwired: 6 in]
              }
              event "Ie limit [mA]:": Value Change {
                n202 = event-data() -> ("NewVal"=w431:dbl)  [unwired: 1 in, 5 out]
                n203 = Multiply(x=w431, y=10.0) -> (x*y=w433:dbl)
                n204 = To Unsigned Word Integer(number=w433) -> (unsigned 16bit integer=w430:u16)
                n205 = call-dynamic "Write Single Holding Register.vi"("error in (no error)"=w434, "holding register value"=w430, "address"=u16 55, "Modbus master in"=w435) -> ("error out"=w436:errorcluster, "Modbus master out"=w437:refnum<class "Modbus Master.lvclass">)  [unwired: 6 in]
              }
              event "Ue limit [V]:": Value Change {
                n206 = event-data() -> ("NewVal"=w440:dbl)  [unwired: 1 in, 5 out]
                n207 = Multiply(x=w440, y=10.0) -> (x*y=w442:dbl)
                n208 = To Unsigned Word Integer(number=w442) -> (unsigned 16bit integer=w439:u16)
                n209 = call-dynamic "Write Single Holding Register.vi"("error in (no error)"=w443, "holding register value"=w439, "address"=u16 56, "Modbus master in"=w444) -> ("error out"=w445:errorcluster, "Modbus master out"=w446:refnum<class "Modbus Master.lvclass">)  [unwired: 6 in]
              }
              event "Target Ue [V]:": Value Change {
                n210 = event-data() -> ("NewVal"=w449:dbl)  [unwired: 1 in, 5 out]
                n211 = Multiply(x=w449, y=10.0) -> (x*y=w451:dbl)
                n212 = To Unsigned Word Integer(number=w451) -> (unsigned 16bit integer=w448:u16)
                n213 = call-dynamic "Write Single Holding Register.vi"("error in (no error)"=w452, "holding register value"=w448, "address"=u16 61, "Modbus master in"=w453) -> ("error out"=w454:errorcluster, "Modbus master out"=w455:refnum<class "Modbus Master.lvclass">)  [unwired: 6 in]
              }
              event "Target Ic [A]:": Value Change {
                n214 = event-data() -> ("NewVal"=w458:dbl)  [unwired: 1 in, 5 out]
                n215 = Multiply(x=w458, y=100.0) -> (x*y=w460:dbl)
                n216 = To Unsigned Word Integer(number=w460) -> (unsigned 16bit integer=w457:u16)
                n217 = call-dynamic "Write Single Holding Register.vi"("error in (no error)"=w461, "holding register value"=w457, "address"=u16 58, "Modbus master in"=w462) -> ("error out"=w463:errorcluster, "Modbus master out"=w464:refnum<class "Modbus Master.lvclass">)  [unwired: 6 in]
              }
              event "Heating Mode:": Value Change {
                n218 = event-data() -> ("NewVal"=w467:bool)  [unwired: 1 in, 5 out]
                n219 = Boolean To (0,1)(Boolean=w467) -> (0, 1=w466:i16)
                n220 = To Unsigned Word Integer(number=w466) -> (unsigned 16bit integer=w468:u16)
                n221 = call-dynamic "Write Single Holding Register.vi"("error in (no error)"=w469, "holding register value"=w468, "address"=u16 22, "Modbus master in"=w470) -> ("error out"=w471:errorcluster, "Modbus master out"=w472:refnum<class "Modbus Master.lvclass">)  [unwired: 6 in]
              }
              event "Regulation TYpe": Value Change {
                n222 = event-data() -> ("NewVal"=w475:bool)  [unwired: 1 in, 5 out]
                n223 = Boolean To (0,1)(Boolean=w475) -> (0, 1=w474:i16)
                n224 = To Unsigned Word Integer(number=w474) -> (unsigned 16bit integer=w476:u16)
                n225 = call-dynamic "Write Single Holding Register.vi"("error in (no error)"=w477, "holding register value"=w476, "address"=u16 21, "Modbus master in"=w478) -> ("error out"=w479:errorcluster, "Modbus master out"=w480:refnum<class "Modbus Master.lvclass">)  [unwired: 6 in]
              }
              event "PID Output:": Value Change {
                n226 = event-data() -> ("NewVal"=w483:bool)  [unwired: 1 in, 5 out]
                n227 = Boolean To (0,1)(Boolean=w483) -> (0, 1=w482:i16)
                n228 = To Unsigned Word Integer(number=w482) -> (unsigned 16bit integer=w484:u16)
                n229 = call-dynamic "Write Single Holding Register.vi"("error in (no error)"=w485, "holding register value"=w484, "address"=u16 57, "Modbus master in"=w486) -> ("error out"=w487:errorcluster, "Modbus master out"=w488:refnum<class "Modbus Master.lvclass">)  [unwired: 6 in]
              }
              event "Target Temp:": Value Change {
                n230 = event-data() -> ("NewVal"=w506:dbl)  [unwired: 1 in, 5 out]
                n231 = local read "Temp. unit:"() -> (w490:u16)
                n232 = Add(x=w506, y=273.15) -> (x+y=w492:dbl)
                n233 = Equal To 0?(x=w490) -> (x = 0?=w493:bool)
                n234 = Select(t=w492, s=w493, f=w506) -> (s? t:f=w491:dbl)
                n235 = Multiply(x=w491, y=100.0) -> (x*y=w500:dbl)
                n236 = To Long Integer(number=w500) -> (32bit integer=w499:i32)
                n237 = Split Number(x=w499) -> (hi(x)=w498:u16, lo(x)=w497:u16)
                n238 = Build Array(w498, w497) -> (w495:u16[])
                n239 = call-dynamic "Write Multiple Holding Registers.vi"("error in (no error)"=w504, "holding register values"=w495, "starting address"=u16 14 ("address"), "Modbus master in"=w505) -> ("error out"=w502:errorcluster, "Modbus master out"=w503:refnum<class "Modbus Master.lvclass">)  [unwired: 6 in]
              }
              event "Target Ramp:": Value Change {
                n240 = event-data() -> ("NewVal"=w516:dbl)  [unwired: 1 in, 5 out]
                n241 = Multiply(x=w516, y=10.0) -> (x*y=w509:dbl)
                n242 = To Word Integer(number=w509) -> (16bit integer=w508:i16)
                n243 = Build Array(w508) -> (w507:i16[])
                n244 = call-dynamic "Write Multiple Holding Registers.vi"("error in (no error)"=w512, "holding register values"=w507, "starting address"=u16 43 ("address"), "Modbus master in"=w513) -> ("error out"=w514:errorcluster, "Modbus master out"=w515:refnum<class "Modbus Master.lvclass">)  [unwired: 6 in]
              }
            }
            n245 = local read "Remote:"() -> (w267:bool)
            n246 = case shown="True" w267 {
              tunnel: w272 -> [w286 w293]
              tunnel: [w286 w292] -> w271
              tunnel: "Lock Button" -> [_ w290]
              tunnel: w270 -> [w285 w288]
              tunnel: [w285 w287] -> w269
              frame False {
              }
              frame True {
                n247 = Boolean To (0,1)(Boolean=w290) -> (0, 1=w289:i16)
                n248 = call-dynamic "Write Single Holding Register.vi"("error in (no error)"=w288, "holding register value"=w289, "address"=1000 ("index"), "Modbus master in"=w293) -> ("error out"=w287:errorcluster, "Modbus master out"=w292:refnum<class "Modbus Master.lvclass">)  [unwired: 6 in]
              }
            }
          }
        }
        n249 = case shown="True" "Auto PID control:" {
          tunnel: "PID manual setting" -> [_ w599]
          tunnel: "PID auto tab" -> [w588 _]
          tunnel: [w579 w594] -> w168
          tunnel: [w578 w593] -> w167
          tunnel: [w577 w592] -> w166
          tunnel: w160 -> [w581 _]
          tunnel: [w575 0] -> w161
          frame False {
            n250 = Decimal String To Number(string=w588, default (0L)=0.0) -> (number=w583:dbl[][])  [unwired: 1 in, 1 out]
            n251 = Delete From Array(array=w583, index (col)=0 ("disabled index (col)")) -> (deleted portion=w580:dbl[], array with subset deleted=w582:dbl[][])  [unwired: 2 in]
            n252 = Threshold 1D Array(2:w581, 3:w580) -> (0:w576:dbl)  [unwired: 1 in]
            n253 = To Long Integer(number=w576) -> (32bit integer=w575:i32)
            n254 = Index Array(array=w582, index (row)=w575, index (col)=1 ("disabled index (col)")) -> (element=w578:dbl)
            n255 = Index Array(array=w582, index (row)=w575, index (col)=2 ("disabled index (col)")) -> (element=w577:dbl)
            n256 = Index Array(array=w582, index (row)=w575, index (col)=0 ("disabled index (col)")) -> (element=w579:dbl)
          }
          frame True {
            w595 = 0 ("disabled index (col)")
            n257 = Decimal String To Number(string=w599, default (0L)=0.0) -> (number=w591:dbl[][])  [unwired: 1 in, 1 out]
            n258 = Index Array(array=w591, index (row)=w595, index (col)=1 ("disabled index (col)")) -> (element=w593:dbl)
            n259 = Index Array(array=w591, index (row)=w595, index (col)=2 ("disabled index (col)")) -> (element=w592:dbl)
            n260 = Index Array(array=w591, index (row)=w595, index (col)=w595) -> (element=w594:dbl)
          }
        }
        "New P:" <- w168
        "New I:" <- w167
        "New D:" <- w166
        n261 = Bundle By Name(cluster=T5 {"Row"=0, "Column"=0} ("Selection Start"), "Row"=w161) -> (w162:T5)
        n262 = property on="PID auto tab" class="Tbl (strict)"("Selection Color"=u32 16860, "Selection Size"=T5 {"Row"=1, "Column"=4}, "Selection Start"=w162) -> ()  [unwired: 2 in, 2 out]
        n263 = Rotate 1D Array(1:w141, 2:1 ("n")) -> (0:w139:dbl[])
        n264 = Replace Array Subset(array=w139, new element=w128) -> (w138:dbl[])  [unwired: 1 in]
        n265 = Index Array(array=w138, index #1=0 ("n"), index #2=19 ("n")) -> (element #1=w134:dbl, element #2=w135:dbl)
        n266 = local read "Text Ring 3"() -> (w130:u16)
        "Text Ring 5" <- w130
        n267 = Subtract(x=w134, y=w135) -> (x-y=w133:dbl)
        n268 = Divide(x=w133, y=10.0) -> (x/y=w131:dbl)
        n269 = case shown="0, Default" w130 {
          tunnel: w131 -> [w172 w175 w179]
          tunnel: [w172 w173 w176] -> w129
          frame 0, Default {
            # "C/s"
          }
          frame 1 {
            # "C/m"
            n270 = Multiply(x=w175, y=60.0) -> (x*y=w173:dbl)
          }
          frame 2 {
            w177 = 60.0 ("y")
            # "C/h"
            n271 = Multiply(x=w179, y=w177) -> (x*y=w178:dbl)
            n272 = Multiply(x=w178, y=w177) -> (x*y=w176:dbl)
          }
        }
        "Act. Ramp:" <- w129
      }
      n273 = Compound Arithmetic op=AND(w116) -> (w125:bool)
      n274 = call-dynamic "Write Single Holding Register.vi"("error in (no error)"=w119, "holding register value"=u16 1, "address"=u16 71, "Modbus master in"=w120) -> ("error out"=w117:errorcluster, "Modbus master out"=w118:refnum<class "Modbus Master.lvclass">)  [unwired: 6 in]
      n275 = local write "stopped_loops"(w125) -> ()
      n276 = call-dynamic "Close.vi"("error in (no error)"=w117, "Modbus master in"=w118) -> ("error out"=w109:errorcluster)  [unwired: 9 in]
      n277 = call <vilib>:"Clear Errors.vi"("error in (no error)"=w109) -> ()  [unwired: 5 in, 2 out]
    }
    frame #2 {
      w613 = "HEAT3 PID manual tab"  # Key 3
      w619 = "HEAT3 PID tab 1"  # Key 2
      w609 = "Section 2"
      w621 = "HEAT3 Path"  # Key 1
      n278 = local read "PID manual setting"() -> (w611:string[][])
      n279 = local read "PID auto tab"() -> (w616:string[][])
      n280 = local read "Address:"() -> (w620:string)
      n281 = call <vilib>:"Application Directory.vi"() -> ("Application Directory"=w607:path)
      n282 = Build Path(base path=w607, name or relative path="TDS Configuration File.ini") -> (appended path=w606:path)
      n283 = Array To Spreadsheet String(array=w616, 3:"%s" ("format string")) -> (spreadsheet string=w618:string)  [unwired: 1 in]
      n284 = Array To Spreadsheet String(array=w611, 3:"%s" ("format string")) -> (spreadsheet string=w610:string)  [unwired: 1 in]
      n285 = Delete(path (use dialog)=w606) -> (deleted path=w624:path)  [unwired: 4 in, 2 out]
      n286 = call <vilib>:"Open Config Data.vi"("configuration file path"=w624) -> ("error out"=w622:errorcluster, "refnum"=w623:T7)  [unwired: 2 in, 7 out]
      n287 = call-poly <vilib>:"Write Key.vi"("section"="Section 1", "error in (no error)"=w622, "value"=w620, "key"=w621, "refnum"=w623) -> ("error out"=w602:errorcluster, "refnum out"=w603:T7)  [unwired: 1 in, 4 out]
      n288 = call-poly <vilib>:"Write Key.vi"("section"=w609, "error in (no error)"=w602, "value"=w618, "key"=w619, "refnum"=w603) -> ("error out"=w614:errorcluster, "refnum out"=w615:T7)  [unwired: 1 in, 4 out]
      n289 = call-poly <vilib>:"Write Key.vi"("section"=w609, "error in (no error)"=w614, "value"=w610, "key"=w613, "refnum"=w615) -> ("error out"=w600:errorcluster, "refnum out"=w601:T7)  [unwired: 1 in, 4 out]
      n290 = call <vilib>:"Close Config Data.vi"("error in (no error)"=w600, "refnum"=w601) -> ("error out"=w604:errorcluster)  [unwired: 1 in, 8 out]
      n291 = call <vilib>:"Clear Errors.vi"("error in (no error)"=w604) -> ()  [unwired: 5 in, 2 out]
    }
  }
  "Connected:" <- w2
  "Comunication error:" <- w2
